vi "IsGUIRunning.vi"(6 "TimeoutInMs(0)":i32, 8 "ErrorIn":errorcluster, 11 "ReferenceIn":refnum<class "TraceWindow.lvclass">) -> (0 "ErrorOut":errorcluster, 1 "Running":bool, 3 "ReferenceOut":refnum<class "TraceWindow.lvclass">)   [LabVIEW 2021, in "TraceWindow.lvlib" / "TraceWindow.lvclass"]
uses:
  TraceWindow.lvclass
  TraceWindow.lvclass/TraceWindow.ctl
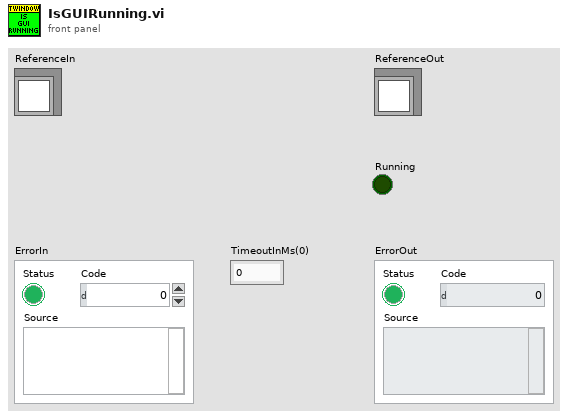
[diagram p1: front panel]
types:
  T1 = typedef "TraceWindow.lvlib/TraceWindow.lvclass/ObjectAttributes.ctl" = cluster{"Interfaces":cluster{"Dummys":refnum<class>}, "Locals":cluster{"MainGUIActive":refnum<queue>, "TraceQueue":refnum<queue>}, "Persistent":cluster{"OpenAtClosure":bool, "BufferSize":i32, "Startup":cluster{"OpenAtStartUp":bool, "OpenMinimized":bool}}}
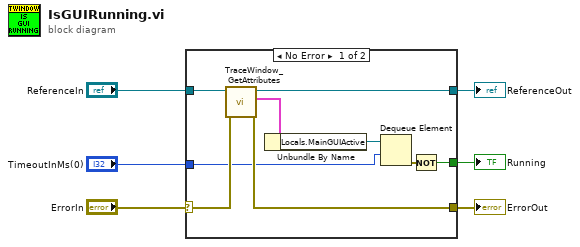
[diagram p0: block diagram]
diagram:
  n1 = case shown="No Error" "ErrorIn" {
    selector: "ErrorIn" -> [w15 w17]
    tunnel: [w13 w17] -> w5
    tunnel: [w10 w16] -> w3
    tunnel: "ReferenceIn" -> [w11 w16]
    tunnel: [w9 _] -> w2
    tunnel: "TimeoutInMs(0)" -> [w7 _]
    frame No Error {
      n2 = call "TraceWindow_GetAttributes.vi"("ErrorIn"=w15, "ReferenceIn"=w11) -> ("ErrorOut"=w13:errorcluster, "Data"=w12:T1, "ReferenceOut"=w10:refnum<class "TraceWindow.lvclass">)  [unwired: 6 in, 1 out]
      n3 = Unbundle By Name(w12) -> ("Locals.MainGUIActive"=w8:refnum<queue>)
      n4 = Dequeue Element(queue=w8, timeout in ms (-1)=w7) -> (error out=w14:errorcluster)  [unwired: 1 in, 3 out]
      n5 = Not(x=w14) -> (.not. x?=w9:bool)
    }
    frame Error {
    }
  }
  "ErrorOut" <- w5
  "ReferenceOut" <- w3
  "Running" <- w2
